vi "Shooter Motor Control.vi"(6 "Filter Strength":dbl(slide) scale=0.0..1.0, 8 "Parallel Cluster":T13, 10 "CounterDevRef":T8, 11 "MotorControlDevRef":T1) -> ()   [LabVIEW 2012]
uses:
  <vilib>/Rock Robotics/WPI/Joystick/WPI_JoystickDevRef.ctl
  <vilib>/Rock Robotics/WPI/Joystick/WPI_JoystickDeviceEnum.ctl
  <vilib>/Rock Robotics/WPI/RobotDrive/WPI_RobotDriveDevRef.ctl
  <vilib>/Rock Robotics/WPI/MotorControl/WPI_MotorControlDeviceRef.ctl
  <vilib>/Rock Robotics/SystemInterfaces/Typedef/FPGA_TypedefDigitalModule.ctl
  <vilib>/Rock Robotics/SystemInterfaces/DIO/FPGA_DIOPWMChannel.ctl
  <vilib>/Rock Robotics/WPI/PWM/WPI_PWMDeadband.ctl
  <vilib>/Rock Robotics/WPI/CAN/Jaguar/SubVIs/WPI_CANJaguar_ControlMode.ctl
  <vilib>/Rock Robotics/WPI/PWM/WPI_PWMTransform_ConPane.ctl
  <vilib>/Rock Robotics/WPI/Counter/WPI_CounterDevRef.ctl
  <vilib>/Rock Robotics/SystemInterfaces/Counter/FPGA_CounterCtrSystemIndex.ctl
  <vilib>/Platform/TimedLoop/XDataNode/timing_clust.ctl
  <vilib>/Platform/TimedLoop/XDataNode/nitl_modes.ctl
  <vilib>/Platform/TimedLoop/XDataNode/wakeup.ctl
  Robot Global Data.vi
  <vilib>/Platform/TimedLoop/XDataNode/XDataNode.xnode
  <vilib>/Platform/TimedLoop/XDataNode/XDNodeRunTimeDep.lvlib
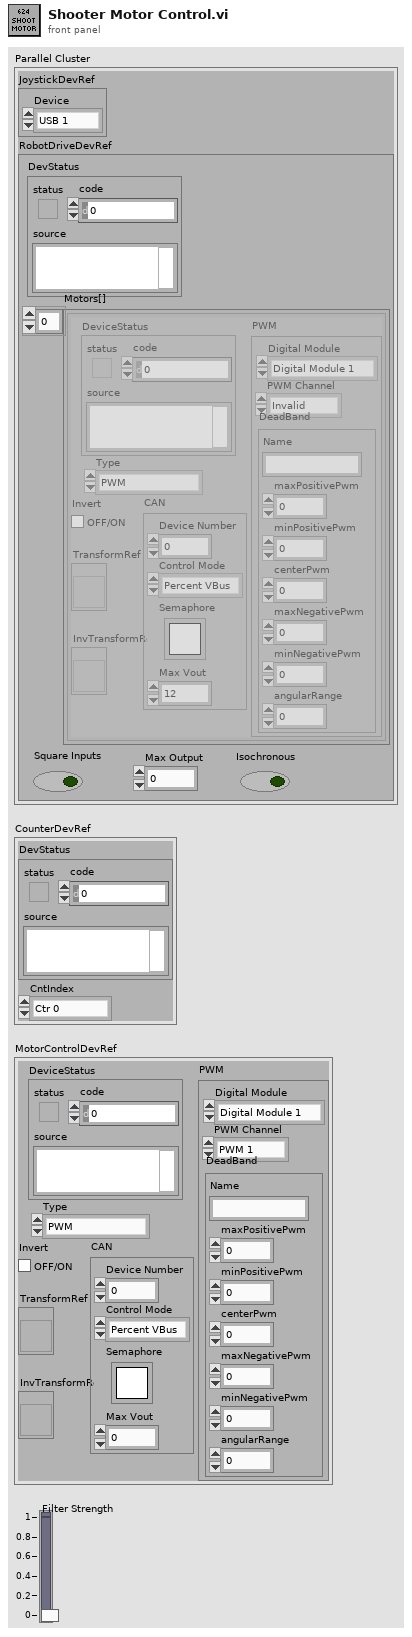
[diagram p1: front panel]
types:
  T1 = typedef "WPI_MotorControlDeviceRef.ctl" = cluster{"DeviceStatus":errorcluster, "Type":enum16{"PWM", "CAN"}, "PWM":cluster{"Digital Module":T2, "PWM Channel":T3, "DeadBand":T4}, "CAN":cluster{"Device Number":u8, "Control Mode":T5, "Semaphore":T6, "Max Vout":dbl}, "Invert":bool, "TransformRef":T7, "InvTransformRef":T7}
  T2 = typedef "FPGA_TypedefDigitalModule.ctl" = enum16{"Digital Module 1", "Digital Module 2"}
  T3 = typedef "FPGA_DIOPWMChannel.ctl" = enum8{"PWM 1", "PWM 2", "PWM 3", "PWM 4", "PWM 5", "PWM 6", "PWM 7", "PWM 8", "PWM 9", "PWM 10", "Invalid"}
  T4 = typedef "WPI_PWMDeadband.ctl" = cluster{"Name":string, "maxPositivePwm":i32, "minPositivePwm":i32, "centerPwm":i32, "maxNegativePwm":i32, "minNegativePwm":i32, "angularRange":u16}
  T5 = typedef "WPI_CANJaguar_ControlMode.ctl" = enum8{"Percent VBus", "Current", "Speed", "Position", "Voltage"}
  T6 = typedef "Semaphore RefNum" = refnum<k1>
  T7 = typedef "WPI_PWMTransform_ConPane.ctl" = refnum<vi>
  T8 = typedef "WPI_CounterDevRef.ctl" = cluster{"DevStatus":errorcluster, "CntIndex":T9}
  T9 = typedef "FPGA_CounterCtrSystemIndex.ctl" = enum8{"Ctr 0", "Ctr 1", "Ctr 2", "Ctr 3", "Ctr 4", "Ctr 5", "Ctr 6", "Ctr 7", "Invalid"}
  T10 = typedef "WPI_JoystickDevRef.ctl" = cluster{"Device":T11}
  T11 = typedef "WPI_JoystickDeviceEnum.ctl" = enum16{"USB 1", "USB 2", "USB 3", "USB 4", "Kinect 1", "Kinect 2"}
  T12 = typedef "WPI_RobotDriveDevRef.ctl" = cluster{"DevStatus":errorcluster, "Motors[]":T1[], "Square Inputs":bool, "Max Output":dbl, "Isochronous":bool}
  T13 = cluster{"JoystickDevRef":T10, "RobotDriveDevRef":T12}
  T14 = typedef "XDNodeRunTimeDep.lvlib/timing_clust.ctl" = cluster{"Expected End [f-1]":u64, "Actual End [f-1]":u64, "Finished Late? [f-1]":bool, "Expected End [i-1]":u64, "Actual End [i-1]":u64, "Finished Late? [i-1]":bool, "Expected Start [i]":u64, "Actual Start [i]":u64, "Expected Start [f]":u64, "Actual Start [f]":u64, "Source Name":string, "Structure Name":string, "Period":i64, "Deadline":i64, "Offset":i64, "Start":i64, "Priority":i32, "Timeout":i32, "Mode":T15, "Wakeup Reason":T16, "Error":errorcluster, "Source Type":string, "Secondary Source Type":string, "Global End Time":u64, "Global Start Time":u64, "Frame Duration":u64, "Iteration Duration":u64, "Assigned CPU":i32, "I/O Scan Engine Mode":u32}
  T15 = typedef "XDNodeRunTimeDep.lvlib/nitl_modes.ctl" = enum32{"No Change", "Process missed periods, maintain original phase", "Discard missed periods, maintain original phase", "Process missed periods, ignore original phase", "Discard missed periods, ignore original phase"}
  T16 = typedef "XDNodeRunTimeDep.lvlib/wakeup.ctl" = enum32{"Normal", "Aborted", "Asynchronous wakeup", "Timing source error", "Timed loop error", "Timeout"}
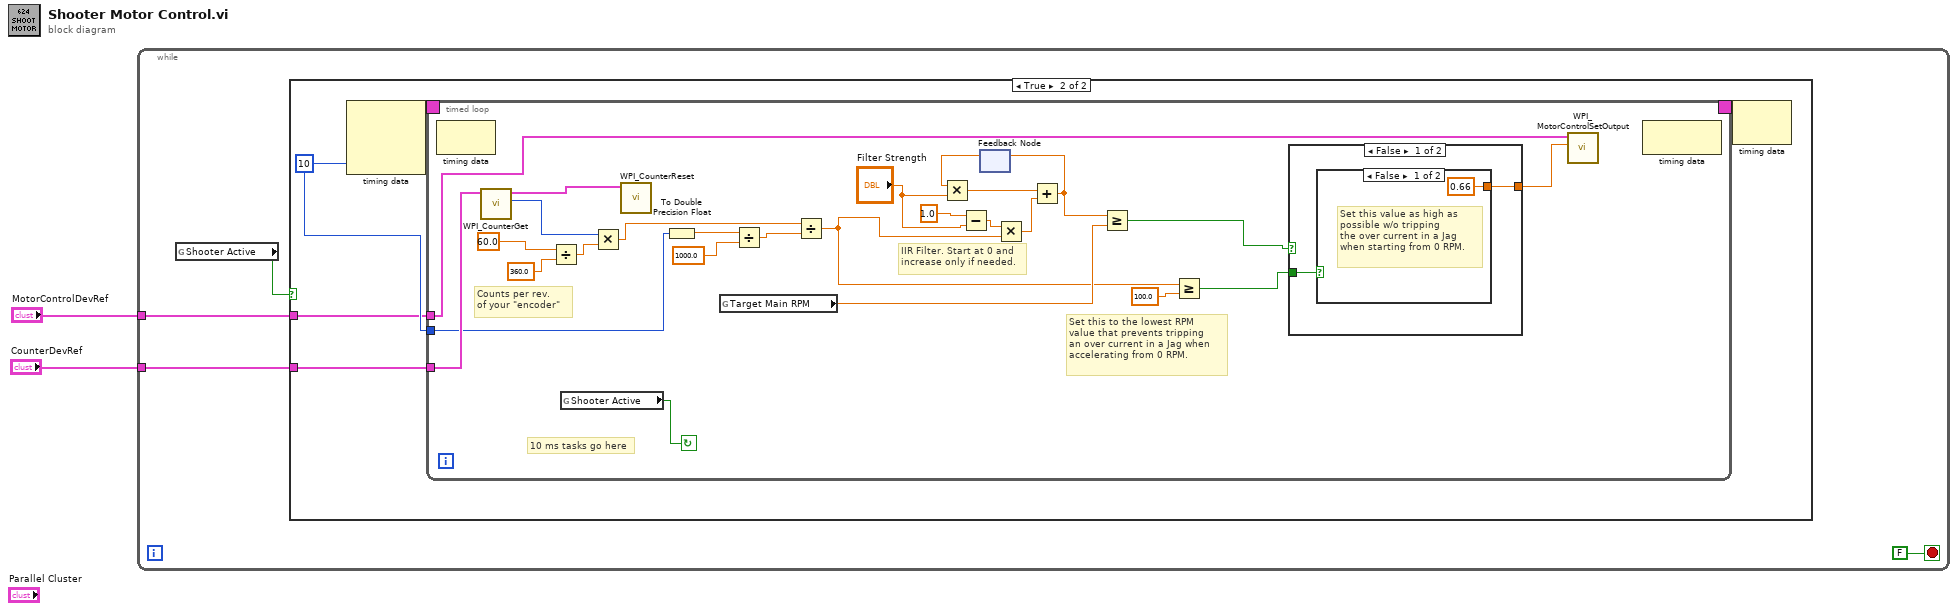
[diagram p0: block diagram]
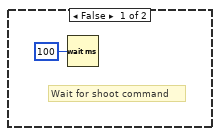
[diagram p2: hidden frame]
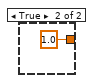
[diagram p3: hidden frame]
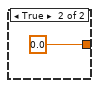
[diagram p4: hidden frame]
diagram:
  n1 = while {
    tunnel: "CounterDevRef" -> [w6]
    tunnel: "MotorControlDevRef" -> [w5]
    stop <- FALSE stop-if-true
    n2 = global read "Robot Global Data.vi" "Shooter Active"() -> (w4:bool)
    n3 = case shown="True" w4 {
      tunnel: w6 -> [_ w9]
      tunnel: w5 -> [_ w8]
      frame False {
        # "Wait for shoot command"
        n4 = Wait (ms)(milliseconds to wait=u32 100) -> ()  [unwired: 1 out]
      }
      frame True {
        w10 = i64 10 ("Period")
        n5 = node-c288(w10) -> (w12:T14)  [unwired: 2 in]
        n6 = timed-loop {
          tunnel: w8 -> [w20]
          tunnel: w9 -> [w38]
          timing: w12 -> [_]
          timing-out: [_] -> w11
          tunnel: w10 -> [w19]
          stop <- w13 continue-if-true
          # "Set this to the lowest RPM \nvalue that prevents tripping\nan over current in a Jag when \naccelerating from 0 RPM."
          # "IIR Filter. Start at 0 and \nincrease only if needed."
          # "Counts per rev. \nof your \"encoder\""
          # "10 ms tasks go here"
          n7 = node-c288() -> ()  [unwired: 1 in, 1 out]
          n8 = call <vilib>:"WPI_CounterGet.vi"("CounterDevRef in"=w38) -> ("Value"=w33:i32, "CounterDevRef out"=w37:T8)  [unwired: 5 in, 4 out]
          n9 = Divide(x=60.0, y=360.0) -> (x/y=w34:dbl)
          n10 = global read "Robot Global Data.vi" "Shooter Active"() -> (w13:bool)
          n11 = Multiply(x=w33, y=w34) -> (x*y=w32:dbl)
          n12 = call <vilib>:"WPI_CounterReset.vi"("CounterDevRef in"=w37) -> ()  [unwired: 9 in, 2 out]
          n13 = To Double Precision Float(number=w19) -> (double precision float=w23:dbl)
          n14 = global read "Robot Global Data.vi" "Target Main RPM"() -> (w25:dbl)
          n15 = Divide(x=w23, y=1000.0) -> (x/y=w24:dbl)
          n16 = Divide(x=w32, y=w24) -> (x/y=w17:dbl)
          n17 = Subtract(x=1.0, y="Filter Strength") -> (x-y=w21:dbl)
          n18 = feedback #1() -> (w31:dbl)  [unwired: 1 in]
          n19 = Multiply(x=w31, y="Filter Strength") -> (x*y=w29:dbl)
          n20 = Multiply(x=w21, y=w17) -> (x*y=w30:dbl)
          n21 = Add(x=w29, y=w30) -> (x+y=w26:dbl)
          n22 = feedback-in #1(w26) -> ()
          n23 = Greater Or Equal?(x=w26, y=w25) -> (x >= y?=w16:bool)
          n24 = Greater Or Equal?(x=w17, y=100.0) -> (x >= y?=w14:bool)
          n25 = case shown="False" w16 {
            tunnel: [w39 0.0] -> w15
            tunnel: w14 -> [w40 _]
            frame False {
              n26 = case shown="False" w40 {
                tunnel: [0.66 1.0] -> w39
                frame False {
                  # "Set this value as high as \npossible w/o tripping\nthe over current in a Jag\nwhen starting from 0 RPM."
                }
                frame True {
                }
              }
            }
            frame True {
            }
          }
          n27 = call <vilib>:"WPI_MotorControlSetOutput.vi"("Output"=w15, "MotorControlDevRef"=w20) -> ()  [unwired: 7 in, 3 out]
          n28 = node-c288() -> ()  [unwired: 1 in, 1 out]
        }
        n29 = node-c288(w11) -> ()  [unwired: 1 out]
      }
    }
  }
